vi "Create Fast Draw Object.vi"(6 "Actual Transform In":T1, 8 "error in (no error)":errorcluster, 9 "Multiplot Representation In":T3, 10 "3D Pie.lvclass in":refnum<class "3D Pie.lvclass">, 11 "Plot Object In":refnum<vi>) -> (0 "error out":errorcluster, 1 "Multiplot Representation Out":T3, 2 "3D Pie.lvclass out":refnum<class "3D Pie.lvclass">, 3 "Plot Object Out":refnum<vi>, 4 "Actual Transform Out":T1)   [LabVIEW 2017, in "3D Pie.lvclass"]
uses:
  <vilib>/Math Plots/3D Math Plots/3D Pie/3D Pie/3D Pie.lvclass
  <vilib>/Math Plots/3D Math Plots/3D Plot/3D Plot/Typedef/Multiplot Representation.ctl
  <vilib>/Math Plots/3D Math Plots/3D Plot/3D Plot/Typedef/Plot Representation.ctl
  <vilib>/Math Plots/3D Math Plots/3D Plot/3D Plot/Typedef/Range Clusters.ctl
  <vilib>/Math Plots/3D Math Plots/3D Plot/3D Plot/Typedef/Mesh Data.ctl
  <vilib>/Math Plots/3D Math Plots/3D Plot/3D Plot/Typedef/Actual Transform.ctl
  <vilib>/Math Plots/3D Math Plots/3D Pie/3D Pie/3D Pie.lvclass/3D Pie.ctl
  <vilib>/Math Plots/3D Math Plots/3D Plot/3D Plot/3D Plot.lvclass
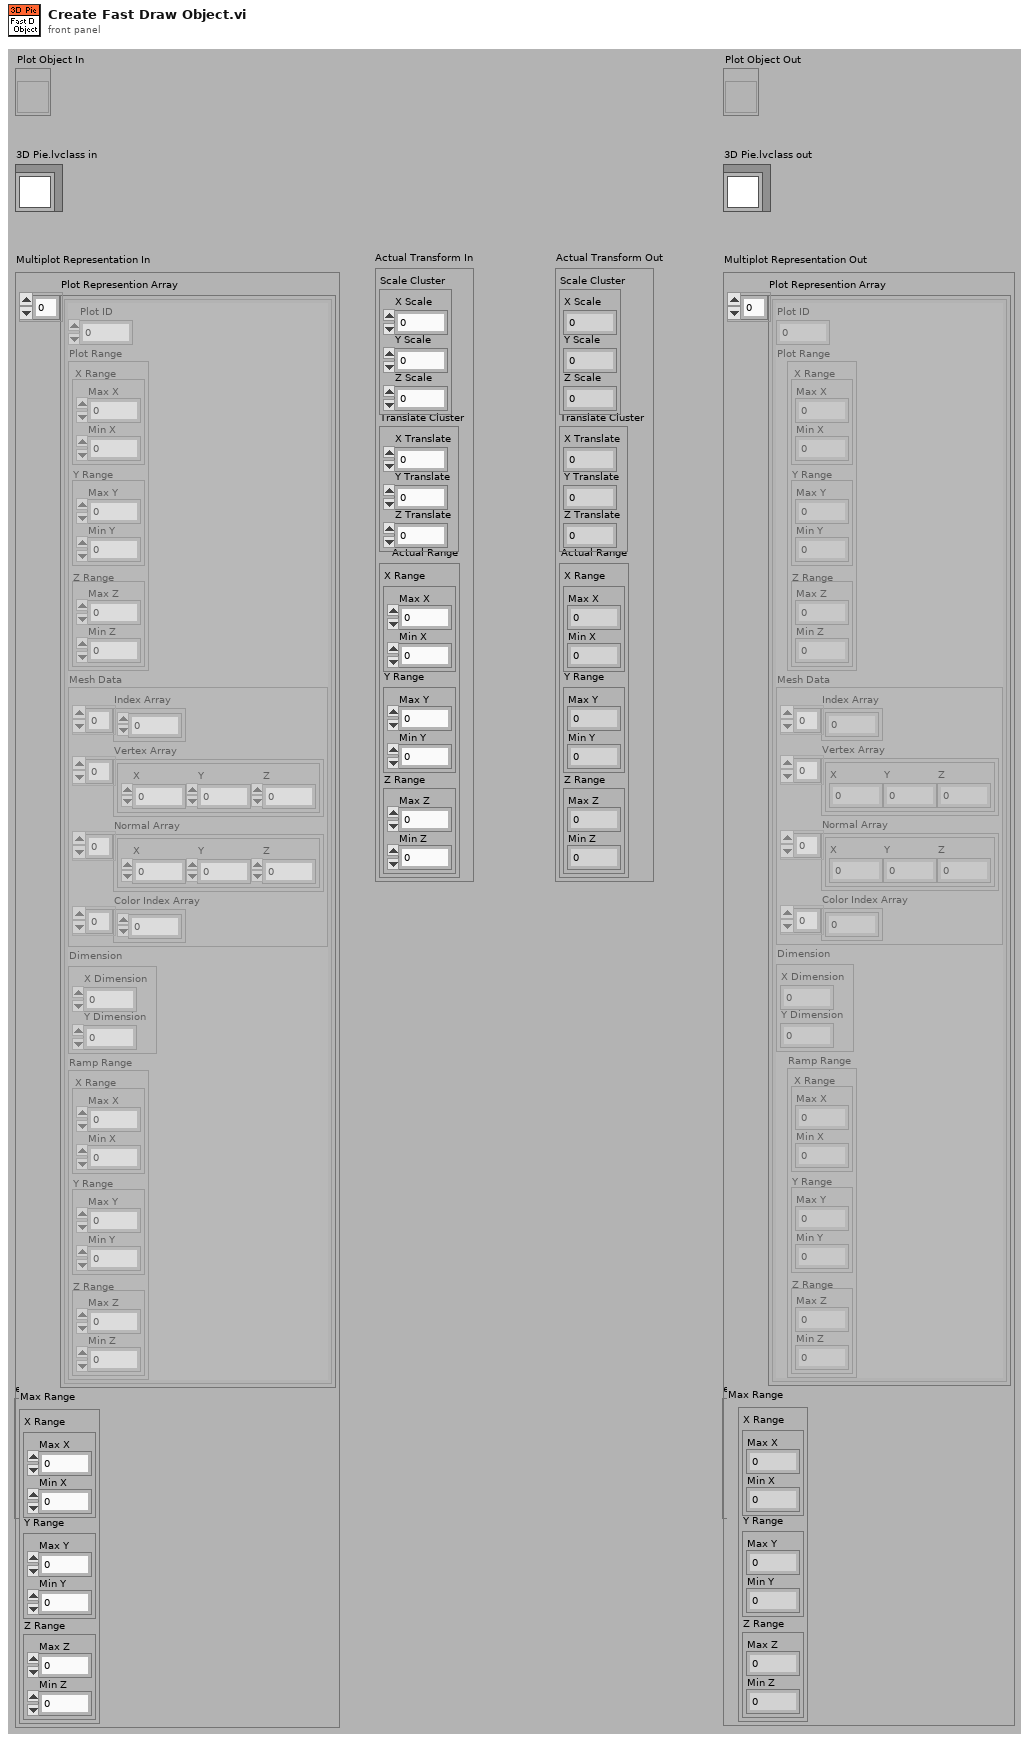
[diagram p1: front panel]
types:
  T1 = typedef "3D Plot.lvclass/Actual Transform.ctl" = cluster{"Scale Cluster":cluster{"X Scale":sgl, "Y Scale":sgl, "Z Scale":sgl}, "Translate Cluster":cluster{"X Translate":sgl, "Y Translate":sgl, "Z Translate":sgl}, "Actual Range":T2}
  T2 = typedef "3D Plot.lvclass/Range Clusters.ctl" = cluster{"X Range":cluster{"Max X":sgl, "Min X":sgl}, "Y Range":cluster{"Max Y":sgl, "Min Y":sgl}, "Z Range":cluster{"Max Z":sgl, "Min Z":sgl}}
  T3 = typedef "3D Plot.lvclass/Multiplot Representation.ctl" = cluster{"Plot Represention Array":T4[], "Max Range":T2}
  T4 = typedef "3D Plot.lvclass/Plot Representation.ctl" = cluster{"Plot ID":i32, "Plot Range":T2, "Mesh Data":T5, "Dimension":cluster{"X Dimension":i32, "Y Dimension":i32}, "Ramp Range":T2}
  T5 = typedef "3D Plot.lvclass/Mesh Data.ctl" = cluster{"Index Array":u32[], "Vertex Array":cluster{"X":sgl, "Y":sgl, "Z":sgl}[], "Normal Array":cluster{"X":sgl, "Y":sgl, "Z":sgl}[], "Color Index Array":i32[]}
  T6 = typedef "3D Pie.lvclass/3D Pie Property Array.ctl" = T7[]
  T7 = typedef "3D Pie.lvclass/3D Pie Property.ctl" = cluster{"General Property":cluster{"Plot Name":string, "Coordinate System":enum16{"Cartesian", "Cylindrical", "Spherical"}, "Opacity":sgl}, "Projection Property":cluster{"Draw XY":bool, "Draw YZ":bool, "Draw XZ":bool}, "Plot Property":cluster{"Line Style":T8, "Line Width":sgl, "Line Color":u32, "Antialiasing":bool}, "Pie Property":cluster{"Pie Height":sgl, "Pie Center":cluster{"X":sgl, "Y":sgl, "Z":sgl}, "Label Mode":enum16{"None", "Show Percentage", "Show String"}, "Label Size":u16, "Label Color":u32, "Color Pair Array":cluster{"Color":u32, "String":string}[], "Slice Offset?":bool}}
  T8 = typedef "3D Plot.lvclass/Line Type.ctl" = enum16{"None", "Solid", "Dash", "Dot", "Dash Dot"}
  T9 = enum16{"Points", "Lines", "Line Strip", "Line Loop", "Triangles", "Triangle Strip", "Triangle Fan", "Quads", "Quad Strip", "Polygon"}
  T10 = cluster{"Draw XY":bool, "Draw YZ":bool, "Draw XZ":bool}
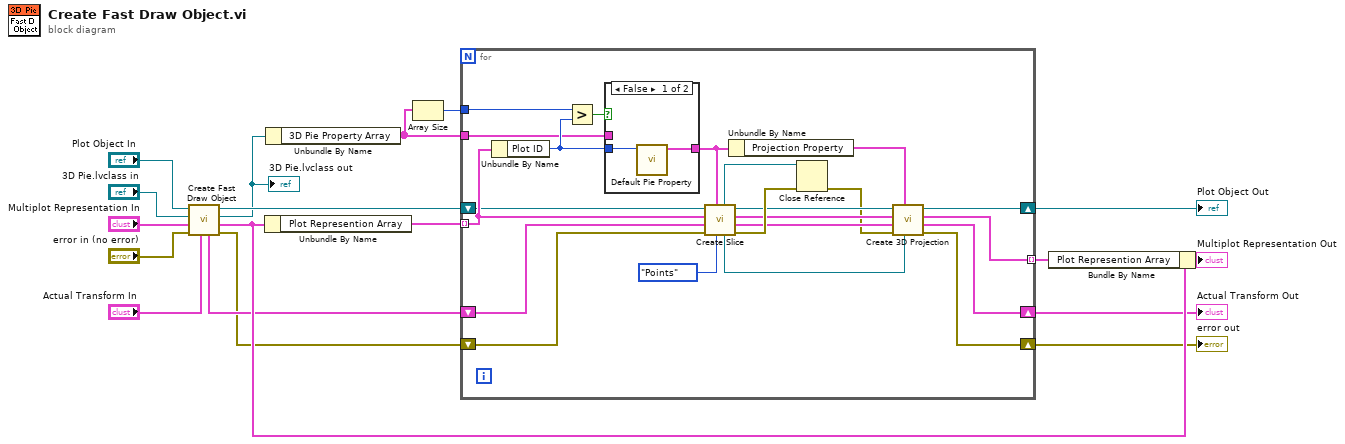
[diagram p0: block diagram]
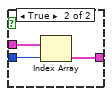
[diagram p2: hidden frame]
diagram:
  n1 = call-parent "Create Fast Draw Object.vi"("Actual Transform In"="Actual Transform In", "error in (no error)"="error in (no error)", "Multiplot Representation In"="Multiplot Representation In", "3D Plot.lvclass in"="3D Pie.lvclass in", "Plot Object In"="Plot Object In") -> ("error out"=w3:errorcluster, "Multiplot Representation Out"=w10:T3, "3D Plot.lvclass out"=w4:refnum<class "3D Pie.lvclass">, "Plot Object Out"=w11:refnum<vi>, "Actual Transform Out"=w9:T1)  [unwired: 2 out]
  "3D Pie.lvclass out" <- w4
  n2 = Unbundle By Name(w10) -> ("Plot Represention Array"=w13:T4[])
  n3 = Unbundle By Name(w4) -> ("3D Pie Property Array"=w1:T6)
  n4 = Array Size(array=w1) -> (size(s)=w2:i32)
  n5 = for {
    tunnel: [w36] -> w12 mode=indexing
    tunnel: w1 -> [w22]
    shift-right: [w35] -> w7
    shift-left: w11 -> [w30]
    shift-right: [w34] -> w5
    shift-left: w3 -> [w29]
    shift-right: [w33] -> w6
    shift-left: w9 -> [w28]
    tunnel: w13 -> [w31] mode=indexing
    tunnel: w2 -> [w24]
    n6 = Unbundle By Name(w31) -> ("Plot ID"=w23:i32)
    n7 = Greater?(x=w24, y=w23) -> (0:w25:bool)
    n8 = case shown="False" w25 {
      tunnel: w22 -> [_ w43]
      tunnel: [w39 w42] -> w21
      tunnel: w23 -> [w40 w41]
      frame False {
        n9 = call <vilib>:"Default Pie Property.vi"("Plot ID"=w40) -> ("Default Property"=w39:T7)  [unwired: 10 out]
      }
      frame True {
        n10 = Index Array(array=w43, index=w41) -> (element=w42:T7)
      }
    }
    n11 = call <vilib>:"Create Slice.vi"("Draw Mode"=T9."Points", "3D Pie Property"=w21, "error in (no error)"=w29, "Plot Representation In"=w31, "Plot Object In"=w30) -> ("error out"=w38:errorcluster, "Plot Representation Out"=w36:T4, "Plot Object Out"=w37:refnum<vi>, "Sector Object Out"=w32:refnum<vi>, "Drawable"=w19:refnum<vi>)  [unwired: 2 out]
    n12 = Unbundle By Name(w21) -> ("Projection Property"=w27:T10)
    n13 = Close Reference(reference=w19, error in (no error)=w38) -> (error out=w20:errorcluster)
    n14 = call <vilib>:"Create 3D Projection.vi"("Sub Object In"=w32, "Projection Property"=w27, "error in (no error)"=w20, "Actual Transform In"=w28, "Plot Object In"=w37) -> ("error out"=w34:errorcluster, "Actual Transform Out"=w33:T1, "Plot Object Out"=w35:refnum<vi>)  [unwired: 1 in, 3 out]
  }
  "error out" <- w5
  "Plot Object Out" <- w7
  "Actual Transform Out" <- w6
  n15 = Bundle By Name(cluster=w10, "Plot Represention Array"=w12) -> (→"Multiplot Representation Out":T3)
